vi "COM_Init.vi"(8 "error in (no error)":errorcluster, 10 "baud rate (9600)":u32, 11 "VISA Refnum in":refnum<visa-resource-name>) -> (0 "error out":errorcluster, 3 "VISA Refnum out":refnum<visa-resource-name>)   [LabVIEW 2020]
uses:
  <vilib>/Instr/_visa.llb/VISA Configure Serial Port (Instr).vi
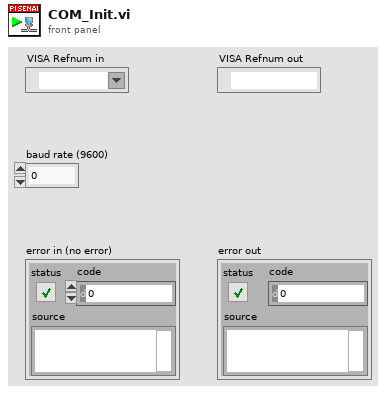
[diagram p1: front panel]
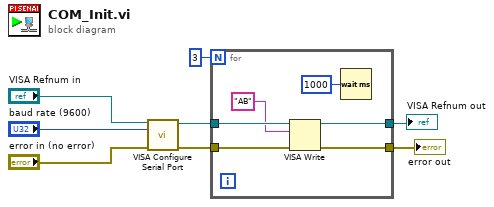
[diagram p0: block diagram]
diagram:
  n1 = call-poly "VISA Configure Serial Port"("VISA resource name"="VISA Refnum in", "baud rate (9600)"="baud rate (9600)", "error in (no error)"="error in (no error)") -> ("VISA resource name out"=w8:refnum<visa-resource-name>, "error out"=w5:errorcluster)  [unwired: 11 in]
  n2 = for {
    N: 3 -> [_]
    tunnel: w5 -> [w13]
    tunnel: [w12] -> w6
    tunnel: [w11] -> w7
    tunnel: w8 -> [w10]
    n3 = VISA Write(VISA resource name=w10, write buffer="AB", error in (no error)=w13) -> (VISA resource name out=w11:refnum<visa-resource-name>, error out=w12:errorcluster)  [unwired: 1 out]
    n4 = Wait (ms)(milliseconds to wait=u32 1000) -> ()  [unwired: 1 out]
  }
  "VISA Refnum out" <- w7
  "error out" <- w6
